vi "funcForGraph.vi"(9 "Ch1":u16(ring) items=["Vin Ch 1", "Vin Ch 2", "Vin Ch 3", "Vin Ch 4", "Vin Ch 5", "Vin Ch 6", "Vin Ch 7", "Vin Ch 8", "Vin Ch 9", "Vin Ch 10", "Vout Ch 1", "Vout Ch 2", "Vout Ch 3", "Vout Ch 4", "Vout Ch 5", "Vout Ch 6", "Vout Ch 7", "Vout Ch 8", "Vout Ch 9", "Vout Ch 10", "Temp1", "Temp 2", "Curren Ch 1", "Curren Ch 2", "Curren Ch 3", "Curren Ch 4", "Curren Ch 5", "Curren Ch 6", "Curren Ch 7", "Curren Ch 8", "Curren Ch 9", "Curren Ch 10"], 10 "UnitType":T1(ring)) -> (2 "curr":enum16{"Vin", "Vout", "Current", "Temp"}(ring))   [LabVIEW 2017]
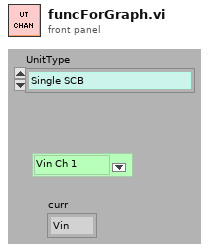
[diagram p1: front panel]
types:
  T1 = enum16{"Single SCB", "Power Rider", "Power Rider&Next10", "HATAL", "DAPH", "Indefinite"}
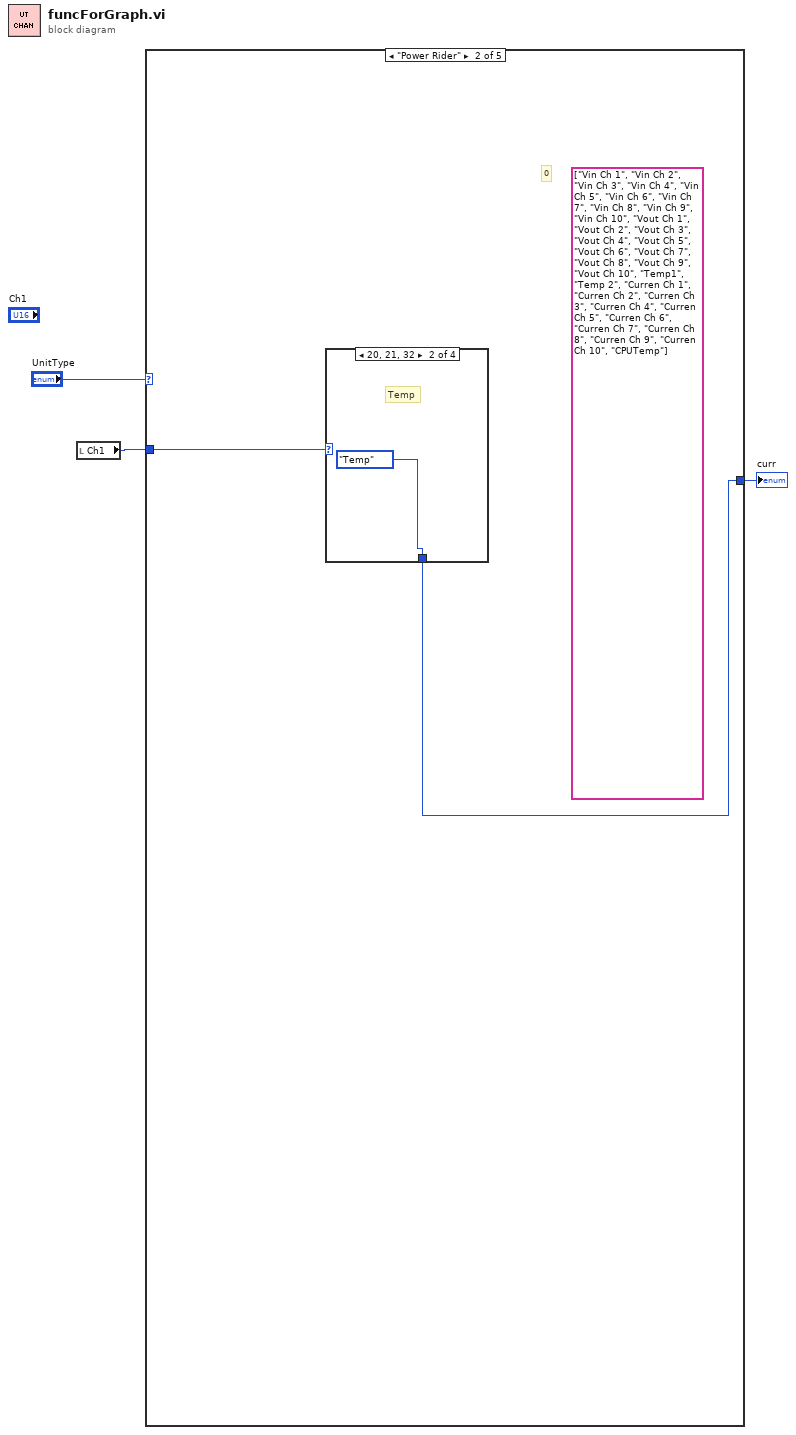
[diagram p0: block diagram]
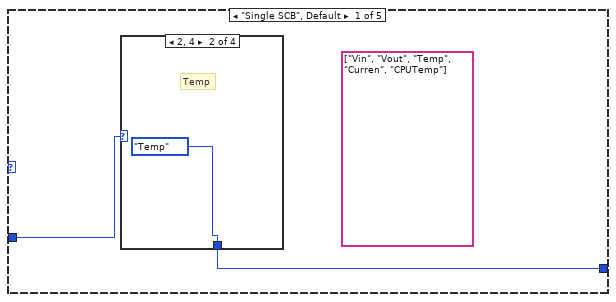
[diagram p2: hidden frame]
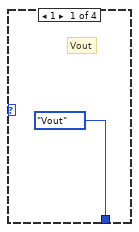
[diagram p3: hidden frame]
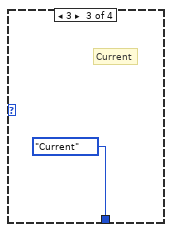
[diagram p4: hidden frame]
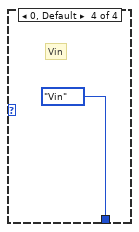
[diagram p5: hidden frame]
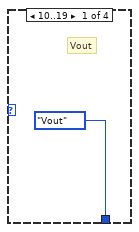
[diagram p6: hidden frame]
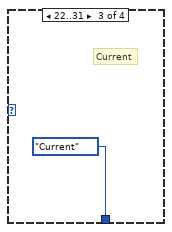
[diagram p7: hidden frame]
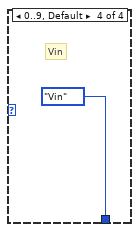
[diagram p8: hidden frame]
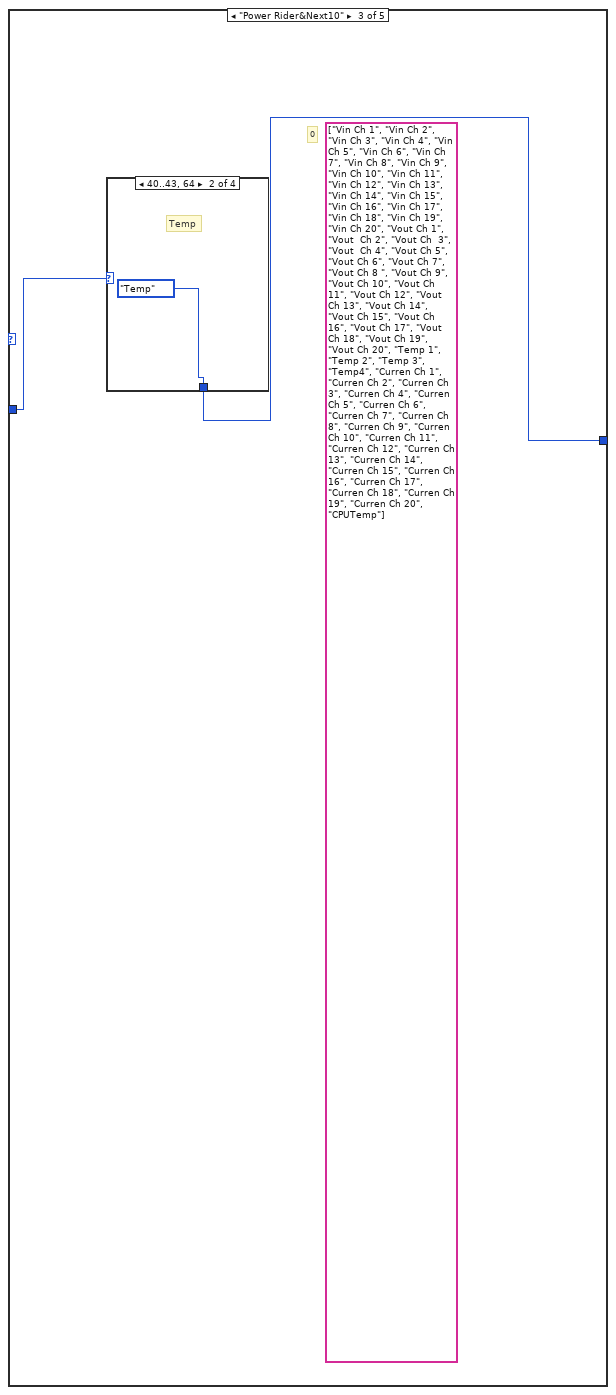
[diagram p9: hidden frame]
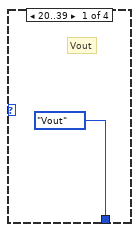
[diagram p10: hidden frame]
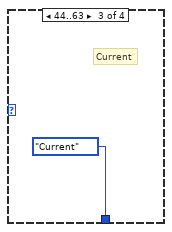
[diagram p11: hidden frame]
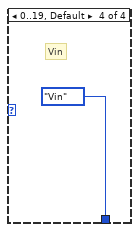
[diagram p12: hidden frame]
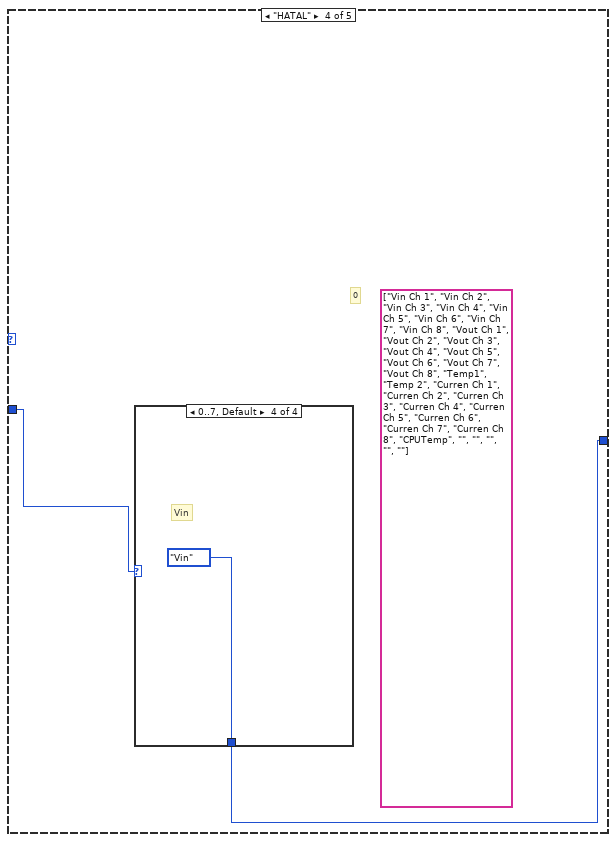
[diagram p13: hidden frame]
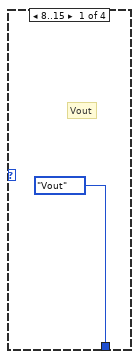
[diagram p14: hidden frame]
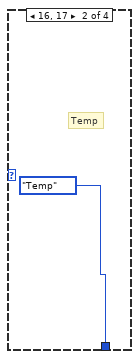
[diagram p15: hidden frame]
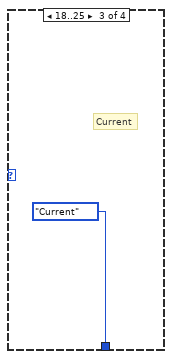
[diagram p16: hidden frame]
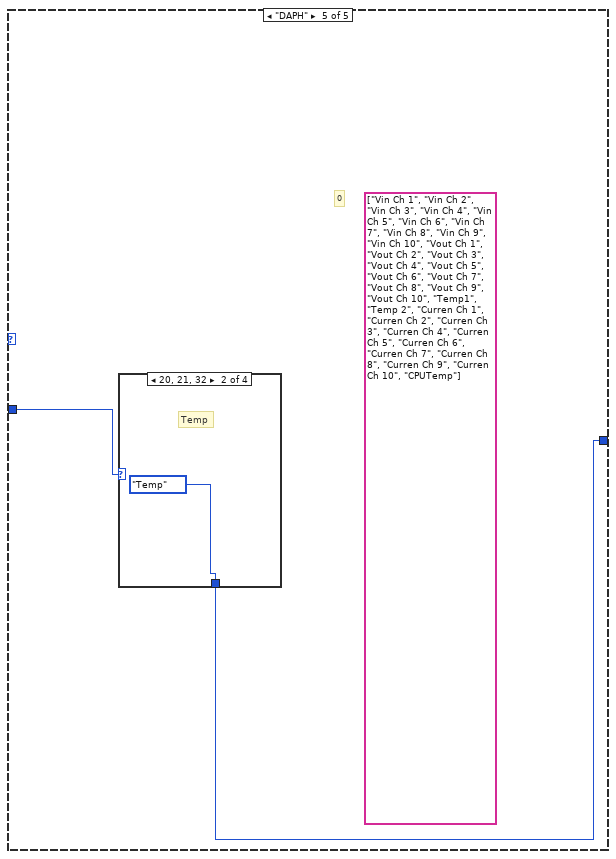
[diagram p17: hidden frame]
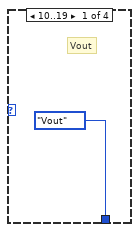
[diagram p18: hidden frame]
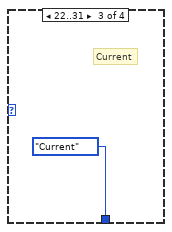
[diagram p19: hidden frame]
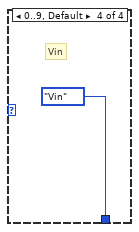
[diagram p20: hidden frame]
diagram:
  n1 = local read "Ch1"() -> (w2:u16)
  n2 = case shown="\"Power Rider\"" "UnitType" {
    tunnel: [w4 w10 w17 w22 w28] -> w3
    tunnel: w2 -> [w5 w11 w16 w23 w29]
    frame "Single SCB", Default {
      (unwired) string[] ["Vin", "Vout", "Temp", "Curren", "CPUTemp"] ("Strings []")
      n3 = case shown="2, 4" w5 {
        tunnel: [enum16{"Vin", "Vout", "Current", "Temp"}."Vout" ("curr") enum16{"Vin", "Vout", "Current", "Temp"}."Temp" ("curr") enum16{"Vin", "Vout", "Current", "Temp"}."Current" ("curr") enum16{"Vin", "Vout", "Current", "Temp"}."Vin" ("curr")] -> w4
        frame 1 {
          # "Vout"
        }
        frame 2, 4 {
          # "Temp"
        }
        frame 3 {
          # "Current"
        }
        frame 0, Default {
          # "Vin"
        }
      }
    }
    frame "Power Rider" {
      (unwired) string[] ["Vin Ch 1", "Vin Ch 2", "Vin Ch 3", "Vin Ch 4", "Vin Ch 5", "Vin Ch 6", "Vin Ch 7", "Vin Ch 8", "Vin Ch 9", "Vin Ch 10", "Vout Ch 1", "Vout Ch 2", "Vout Ch 3", "Vout Ch 4", "Vout Ch 5", "Vout Ch 6", "Vout Ch 7", "Vout Ch 8", "Vout Ch 9", "Vout Ch 10", "Temp1", "Temp 2", "Curren Ch 1", "Curren Ch 2", "Curren Ch 3", "Curren Ch 4", "Curren Ch 5", "Curren Ch 6", "Curren Ch 7", "Curren Ch 8", "Curren Ch 9", "Curren Ch 10", "CPUTemp"] ("Strings []")
      # "31"
      # "22"
      # "20"
      # "21"
      # "19"
      # "10"
      # "9"
      # "0"
      n4 = case shown="20, 21, 32" w11 {
        tunnel: [enum16{"Vin", "Vout", "Current", "Temp"}."Vout" ("curr") enum16{"Vin", "Vout", "Current", "Temp"}."Temp" ("curr") enum16{"Vin", "Vout", "Current", "Temp"}."Current" ("curr") enum16{"Vin", "Vout", "Current", "Temp"}."Vin" ("curr")] -> w10
        frame 10..19 {
          # "Vout"
        }
        frame 20, 21, 32 {
          # "Temp"
        }
        frame 22..31 {
          # "Current"
        }
        frame 0..9, Default {
          # "Vin"
        }
      }
    }
    frame "Power Rider&Next10" {
      (unwired) string[] ["Vin Ch 1", "Vin Ch 2", "Vin Ch 3", "Vin Ch 4", "Vin Ch 5", "Vin Ch 6", "Vin Ch 7", "Vin Ch 8", "Vin Ch 9", "Vin Ch 10", "Vin Ch 11", "Vin Ch 12", "Vin Ch 13", "Vin Ch 14", "Vin Ch 15", "Vin Ch 16", "Vin Ch 17", "Vin Ch 18", "Vin Ch 19", "Vin Ch 20", "Vout Ch 1", "Vout  Ch 2", "Vout Ch  3", "Vout  Ch 4", "Vout Ch 5", "Vout Ch 6", "Vout Ch 7", "Vout Ch 8 ", "Vout Ch 9", "Vout Ch 10", "Vout Ch 11", "Vout Ch 12", "Vout Ch 13", "Vout Ch 14", "Vout Ch 15", "Vout Ch 16", "Vout Ch 17", "Vout Ch 18", "Vout Ch 19", "Vout Ch 20", "Temp 1", "Temp 2", "Temp 3", "Temp4", "Curren Ch 1", "Curren Ch 2", "Curren Ch 3", "Curren Ch 4", "Curren Ch 5", "Curren Ch 6", "Curren Ch 7", "Curren Ch 8", "Curren Ch 9", "Curren Ch 10", "Curren Ch 11", "Curren Ch 12", "Curren Ch 13", "Curren Ch 14", "Curren Ch 15", "Curren Ch 16", "Curren Ch 17", "Curren Ch 18", "Curren Ch 19", "Curren Ch 20", "CPUTemp"] ("Strings []")
      # "63"
      # "44"
      # "43"
      # "40"
      # "39"
      # "20"
      # "19"
      # "0"
      n5 = case shown="40..43, 64" w16 {
        tunnel: [enum16{"Vin", "Vout", "Current", "Temp"}."Vout" ("curr") enum16{"Vin", "Vout", "Current", "Temp"}."Temp" ("curr") enum16{"Vin", "Vout", "Current", "Temp"}."Current" ("curr") enum16{"Vin", "Vout", "Current", "Temp"}."Vin" ("curr")] -> w17
        frame 20..39 {
          # "Vout"
        }
        frame 40..43, 64 {
          # "Temp"
        }
        frame 44..63 {
          # "Current"
        }
        frame 0..19, Default {
          # "Vin"
        }
      }
    }
    frame "HATAL" {
      (unwired) string[] ["Vin Ch 1", "Vin Ch 2", "Vin Ch 3", "Vin Ch 4", "Vin Ch 5", "Vin Ch 6", "Vin Ch 7", "Vin Ch 8", "Vout Ch 1", "Vout Ch 2", "Vout Ch 3", "Vout Ch 4", "Vout Ch 5", "Vout Ch 6", "Vout Ch 7", "Vout Ch 8", "Temp1", "Temp 2", "Curren Ch 1", "Curren Ch 2", "Curren Ch 3", "Curren Ch 4", "Curren Ch 5", "Curren Ch 6", "Curren Ch 7", "Curren Ch 8", "CPUTemp", "", "", "", "", ""] ("Strings []")
      # "25"
      # "18"
      # "16"
      # "17"
      # "15"
      # "8"
      # "7"
      # "0"
      n6 = case shown="0..7, Default" w23 {
        tunnel: [enum16{"Vin", "Vout", "Current", "Temp"}."Vout" ("curr") enum16{"Vin", "Vout", "Current", "Temp"}."Temp" ("curr") enum16{"Vin", "Vout", "Current", "Temp"}."Current" ("curr") enum16{"Vin", "Vout", "Current", "Temp"}."Vin" ("curr")] -> w22
        frame 8..15 {
          # "Vout"
        }
        frame 16, 17 {
          # "Temp"
        }
        frame 18..25 {
          # "Current"
        }
        frame 0..7, Default {
          # "Vin"
        }
      }
    }
    frame "DAPH" {
      (unwired) string[] ["Vin Ch 1", "Vin Ch 2", "Vin Ch 3", "Vin Ch 4", "Vin Ch 5", "Vin Ch 6", "Vin Ch 7", "Vin Ch 8", "Vin Ch 9", "Vin Ch 10", "Vout Ch 1", "Vout Ch 2", "Vout Ch 3", "Vout Ch 4", "Vout Ch 5", "Vout Ch 6", "Vout Ch 7", "Vout Ch 8", "Vout Ch 9", "Vout Ch 10", "Temp1", "Temp 2", "Curren Ch 1", "Curren Ch 2", "Curren Ch 3", "Curren Ch 4", "Curren Ch 5", "Curren Ch 6", "Curren Ch 7", "Curren Ch 8", "Curren Ch 9", "Curren Ch 10", "CPUTemp"] ("Strings []")
      # "31"
      # "22"
      # "20"
      # "21"
      # "19"
      # "10"
      # "9"
      # "0"
      n7 = case shown="20, 21, 32" w29 {
        tunnel: [enum16{"Vin", "Vout", "Current", "Temp"}."Vout" ("curr") enum16{"Vin", "Vout", "Current", "Temp"}."Temp" ("curr") enum16{"Vin", "Vout", "Current", "Temp"}."Current" ("curr") enum16{"Vin", "Vout", "Current", "Temp"}."Vin" ("curr")] -> w28
        frame 10..19 {
          # "Vout"
        }
        frame 20, 21, 32 {
          # "Temp"
        }
        frame 22..31 {
          # "Current"
        }
        frame 0..9, Default {
          # "Vin"
        }
      }
    }
  }
  "curr" <- w3
